vi "Save Transport DAT File 2D.vi"(8 "error in (no error)":errorcluster, 10 "Data (Multiple Row)":dbl[][](array[numeric]), 11 "Control Experiment in":refnum<class "Control Experiment SM.lvclass">) -> (0 "error out":errorcluster, 3 "Control Experiment out":refnum<class "Control Experiment SM.lvclass">)   [LabVIEW 2016, in "Control Experiment SM.lvclass"]
uses:
  Control Experiment SM.lvclass
  <vilib>/Utility/file.llb/Write Delimited Spreadsheet (string).vi
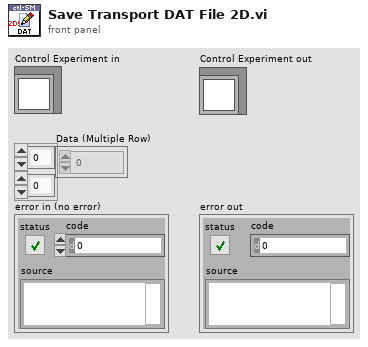
[diagram p1: front panel]
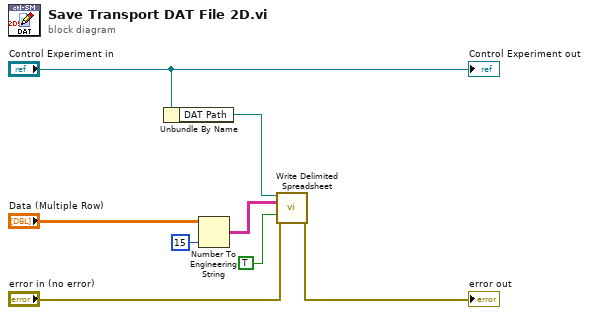
[diagram p0: block diagram]
diagram:
  n1 = Unbundle By Name("Control Experiment in") -> ("DAT Path"=w6:path)
  n2 = Number To Engineering String(2:i16 15 ("precision (6)"), 4:"Data (Multiple Row)") -> (0:w4:string[][])  [unwired: 2 out]
  n3 = call-poly <vilib>:"Write Delimited Spreadsheet.vi"("file path (dialog if empty)"=w6, "2D data"=w4, "append to file? (new file:F)"=TRUE, "error in (no error)"="error in (no error)") -> ("error out"=→"error out":errorcluster)  [unwired: 10 in, 1 out]
  "Control Experiment out" <- "Control Experiment in"
